vi "DEMO using all functions K_S30_VISA.vi"() -> ()   [LabVIEW 2012]
panel:
  in  "Stopp":bool
  out "Configuration read":u8 format="%.0x"
  in  "Configuration write":u8
  in  "Config. Nr.":u8=1
  in  "Coeff write":sgl format="%.6e"
  out "Coeff read":sgl format="%.6e"
  in  "Coeff. Nr.":u8=64
  out "Status":u8 format="%.0b"
  out "Value":sgl format="%.6e"
  in  "Channel 2":enum16{"CH0", "P1", "P2", "T", "TOB1", "TOB2"}(ring)=enum."P1"
  in  "Target Value":sgl format="%.6e"
  in  "Command":T1(ring)
  in  "F73 read Value":bool
  in  "F33 write config":bool
  in  "F31 write Coeff":bool
  out "Actual Address":u8
  in  "New Address":u8
  out "Serial Nr.":u32
  out "Information":T2
  in  "RS-converter: echo":bool=TRUE
  in  "timeout":u32=50
  in  "Baudrate":enum16{"9600", "115200"}(ring)
  in  "VISA":refnum<visa-resource-name>="COM1"
  in  "F32 read config":bool
  in  "F95 zero":bool
  in  "F66 Device Addr":bool
  in  "F69 SN":bool
  in  "F30 read Coeff":bool
  in  "F48 ini":bool
  in  "Close Com":bool
  in  "Open Com":bool
  in  "Online":bool
  out "error":errorcluster
  out "Value":sgl(graph)
  in  "Channel":enum16{"CH0", "P1", "P2", "T", "TOB1", "TOB2"}(ring)=enum."P1"
  in  "Address":u8=250
  # "Communication with KELLER pressure transmitters Series 3.X using LabView\n\nDemo for all low-level VI's using VISA"
  # "ComPort will also be opened, if you change an parameter for the ComPort"
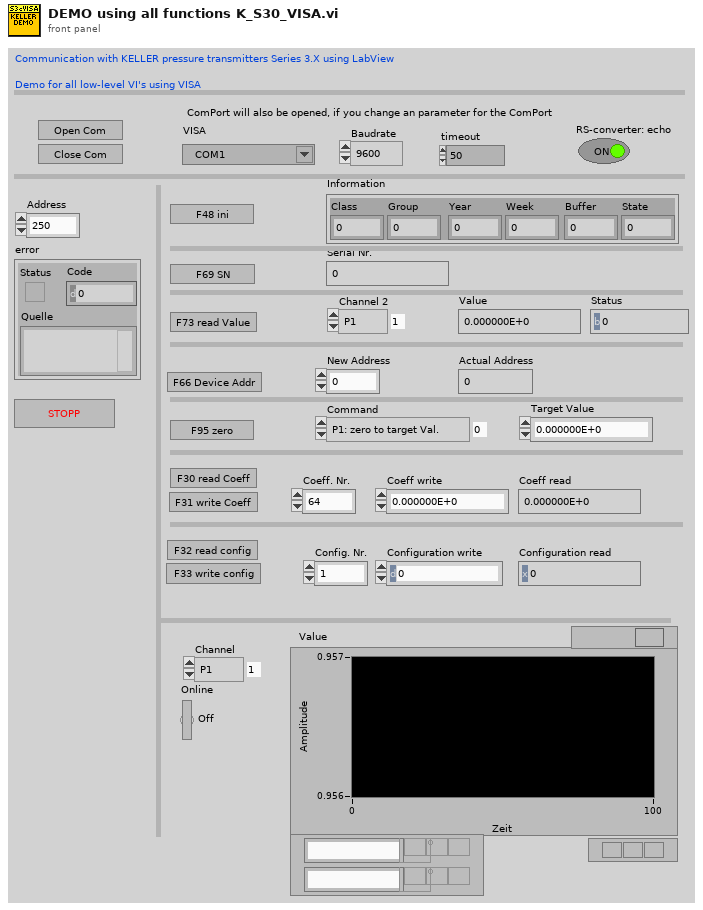
[diagram p1: front panel]
types:
  T1 = enum8{"P1: zero to target Val.", "P1: reset zero", "P2: zero to target Val.", "P2: reset zero", "cmd 4", "cmd 5", "CH0: zero to target Val.", "CH0: reset zero"}
  T2 = cluster{"Class":u8, "Group":u8, "Year":u8, "Week":u8, "Buffer":u8, "State":u8}
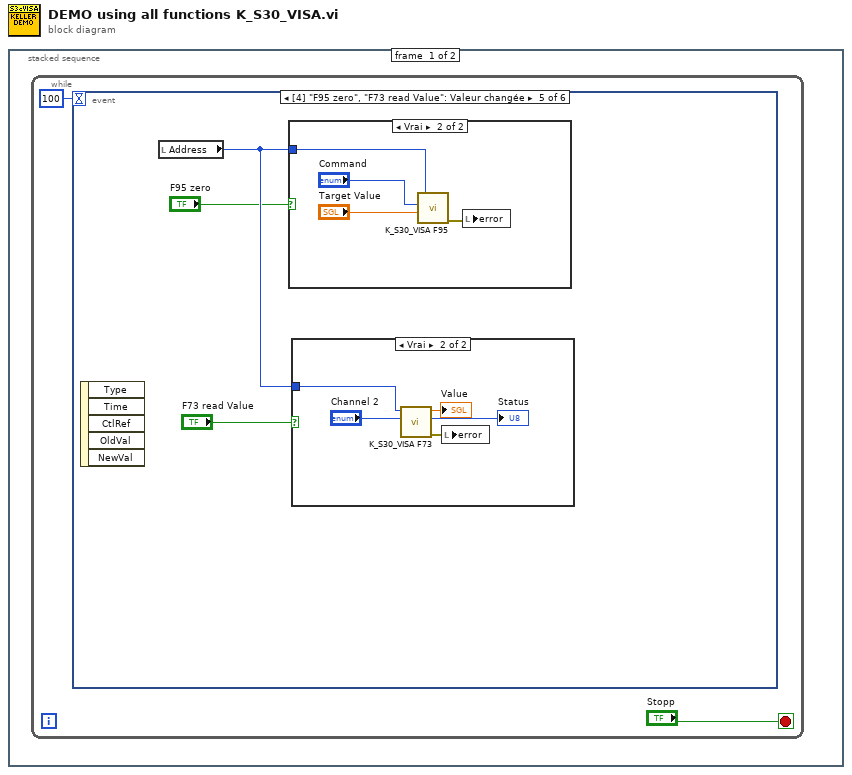
[diagram p0: block diagram]
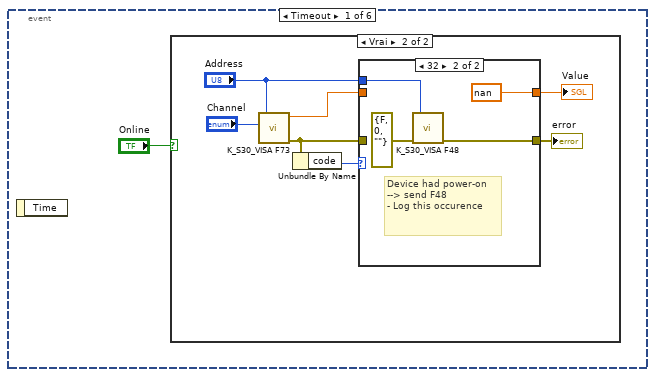
[diagram p2: hidden frame]
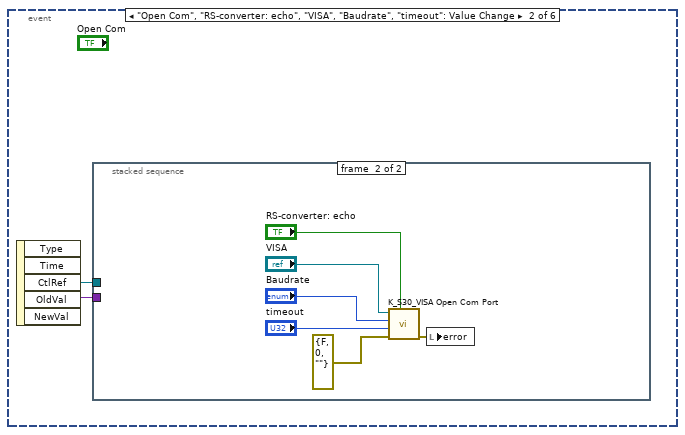
[diagram p5: hidden frame]
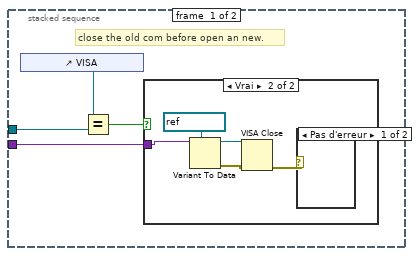
[diagram p6: hidden frame]
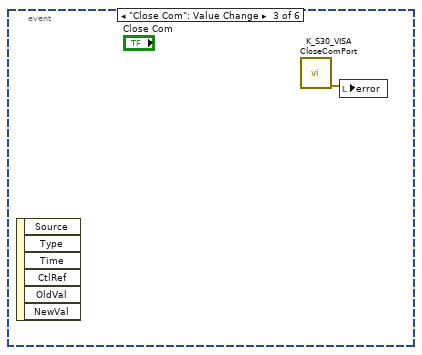
[diagram p9: hidden frame]
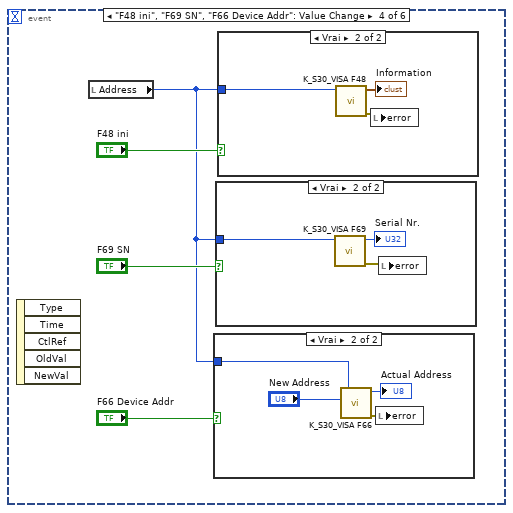
[diagram p10: hidden frame]
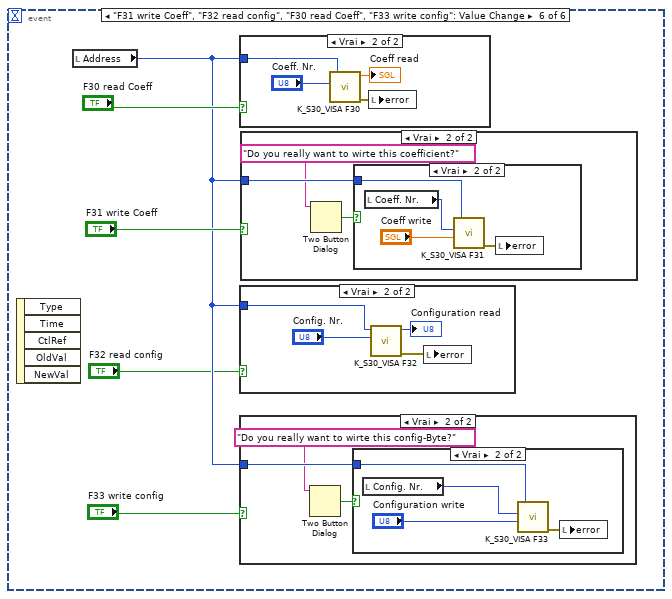
[diagram p16: hidden frame]
diagram:
  n1 = stacked-sequence {
    frame #0 {
      n2 = while {
        stop <- "Stopp" stop-if-true
        n3 = event shown="[4] \"F95 zero\", \"F73 read Value\": Valeur changée" {
          selector: _ -> [_ _ _ _ _ _]
          dyn-events: _ -> [_ _ _ _ _ _]
          timeout: 100 -> [_ _ _ _ _ _]
          event Timeout {
            n4 = event-data() -> ()  [unwired: 1 in, 1 out]
            n5 = case shown="Vrai" "Online" {
              frame False {
              }
              frame True {
                n6 = call "K_S30_VISA F73.vi"("Channel"="Channel", "Address"="Address") -> ("error out"=w7:errorcluster, "Value"=w6:sgl)  [unwired: 3 in, 1 out]
                n7 = Unbundle By Name(w7) -> ("code"=w9:i32)
                n8 = case shown="32" w9 {
                  tunnel: "Address" -> [_ w15]
                  tunnel: w7 -> [w11 _]
                  tunnel: w6 -> [w12 _]
                  tunnel: [w12 sgl nan] -> w5
                  tunnel: [w11 w13] -> w4
                  frame 0, Default {
                  }
                  frame 32 {
                    # "Device had power-on\n--> send F48\n- Log this occurence"
                    n9 = call "K_S30_VISA F48.vi"("error in"=errorcluster {"status"=FALSE, "code"=0, "source"=""}, "Address"=w15) -> ("error out"=w13:errorcluster)  [unwired: 3 in, 2 out]
                  }
                }
                "Value" <- w5
                "error" <- w4
              }
            }
          }
          event "Open Com", "RS-converter: echo", "VISA", "Baudrate", "timeout": Value Change {
            n10 = event-data() -> ("CtlRef"=w18:refnum<vi>, "OldVal"=w17:variant)  [unwired: 1 in, 3 out]
            n11 = stacked-sequence {
              tunnel: w18 -> [w20 _]
              tunnel: w17 -> [w21 _]
              frame #0 {
                # "close the old com before open an new."
                n12 = control-ref of="VISA"() -> (w19:refnum<vi>)
                n13 = Equal?(x=w19, y=w20) -> (x = y?=w22:bool)
                n14 = case shown="Vrai" w22 {
                  tunnel: w21 -> [_ w27]
                  frame False {
                  }
                  frame True {
                    n15 = Variant To Data(type=refnum<visa-resource-name> "COM1" ("VISA resource name"), Variant=w27) -> (data=w25:refnum<visa-resource-name>, error out=w24:errorcluster)  [unwired: 1 in]
                    n16 = VISA Close(VISA resource name=w25, error in (no error)=w24) -> (error out=w23:errorcluster)
                    n17 = case shown="Pas d'erreur" w23 {
                      frame No Error {
                      }
                      frame Error {
                      }
                    }
                  }
                }
              }
              frame #1 {
                n18 = call "K_S30_VISA Open Com Port.vi"("RS-converter:\necho"="RS-converter: echo", "error in (no error)"=errorcluster {"status"=FALSE, "code"=0, "source"=""}, "timeout"="timeout", "Baudrate"="Baudrate", "VISA resource name"="VISA") -> ("error out"=w29:errorcluster)  [unwired: 3 in, 1 out]
                n19 = local write "error"(w29) -> ()
              }
            }
          }
          event "Close Com": Value Change {
            n20 = event-data() -> ()  [unwired: 1 in, 6 out]
            n21 = call "K_S30_VISA CloseComPort.vi"() -> ("Fehlerausgang"=w34:errorcluster)  [unwired: 7 in]
            n22 = local write "error"(w34) -> ()
          }
          event "F48 ini", "F69 SN", "F66 Device Addr": Value Change {
            n23 = event-data() -> ()  [unwired: 1 in, 5 out]
            n24 = local read "Address"() -> (w35:u8)
            n25 = case shown="Vrai" "F66 Device Addr" {
              tunnel: w35 -> [_ w42]
              frame False {
              }
              frame True {
                n26 = call "K_S30_VISA F66.vi"("New Address"="New Address", "Address"=w42) -> ("error out"=w39:errorcluster, "Actual Address"=→"Actual Address":u8)  [unwired: 4 in]
                n27 = local write "error"(w39) -> ()
              }
            }
            n28 = case shown="Vrai" "F69 SN" {
              tunnel: w35 -> [_ w45]
              frame False {
              }
              frame True {
                n29 = call "K_S30_VISA F69.vi"("Address"=w45) -> ("error out"=w43:errorcluster, "Serial Nr."=→"Serial Nr.":u32)  [unwired: 5 in]
                n30 = local write "error"(w43) -> ()
              }
            }
            n31 = case shown="Vrai" "F48 ini" {
              tunnel: w35 -> [_ w46]
              frame False {
              }
              frame True {
                n32 = call "K_S30_VISA F48.vi"("Address"=w46) -> ("error out"=w48:errorcluster, "Information"=→"Information":T2)  [unwired: 4 in, 1 out]
                n33 = local write "error"(w48) -> ()
              }
            }
          }
          event "F95 zero", "F73 read Value": Value Change {
            n34 = event-data() -> ()  [unwired: 1 in, 5 out]
            n35 = local read "Address"() -> (w51:u8)
            n36 = case shown="Vrai" "F95 zero" {
              tunnel: w51 -> [_ w60]
              frame False {
              }
              frame True {
                n37 = call "K_S30_VISA F95.vi"("Target Value"="Target Value", "Command"="Command", "Address"=w60) -> ("error out"=w57:errorcluster)  [unwired: 4 in]
                n38 = local write "error"(w57) -> ()
              }
            }
            n39 = case shown="Vrai" "F73 read Value" {
              tunnel: w51 -> [_ w56]
              frame False {
              }
              frame True {
                n40 = call "K_S30_VISA F73.vi"("Channel"="Channel 2", "Address"=w56) -> ("error out"=w54:errorcluster, "Status"=→"Status":u8, "Value"=→"Value":sgl)  [unwired: 3 in]
                n41 = local write "error"(w54) -> ()
              }
            }
          }
          event "F31 write Coeff", "F32 read config", "F30 read Coeff", "F33 write config": Value Change {
            n42 = event-data() -> ()  [unwired: 1 in, 5 out]
            n43 = local read "Address"() -> (w62:u8)
            n44 = case shown="Vrai" "F30 read Coeff" {
              tunnel: w62 -> [_ w87]
              frame False {
              }
              frame True {
                n45 = call "K_S30_VISA F30.vi"("Coeff. Nr."="Coeff. Nr.", "Address"=w87) -> ("error out"=w85:errorcluster, "Coeff"=→"Coeff read":sgl)  [unwired: 4 in]
                n46 = local write "error"(w85) -> ()
              }
            }
            n47 = case shown="Vrai" "F32 read config" {
              tunnel: w62 -> [_ w76]
              frame False {
              }
              frame True {
                n48 = call "K_S30_VISA F32.vi"("Config. Nr."="Config. Nr.", "Address"=w76) -> ("error out"=w73:errorcluster, "Configuration"=→"Configuration read":u8)  [unwired: 4 in]
                n49 = local write "error"(w73) -> ()
              }
            }
            n50 = case shown="Vrai" "F33 write config" {
              tunnel: w62 -> [_ w68]
              frame False {
              }
              frame True {
                n51 = Two Button Dialog(message="Do you really want to wirte this config-Byte?" ("Nachricht")) -> (T button?=w67:bool)  [unwired: 2 in]
                n52 = case shown="Vrai" w67 {
                  tunnel: w68 -> [_ w72]
                  frame False {
                  }
                  frame True {
                    n53 = local read "Config. Nr."() -> (w70:u8)
                    n54 = call "K_S30_VISA F33.vi"("Configuration"="Configuration write", "Config. Nr."=w70, "Address"=w72) -> ("error out"=w71:errorcluster)  [unwired: 4 in]
                    n55 = local write "error"(w71) -> ()
                  }
                }
              }
            }
            n56 = case shown="Vrai" "F31 write Coeff" {
              tunnel: w62 -> [_ w79]
              frame False {
              }
              frame True {
                n57 = Two Button Dialog(message="Do you really want to wirte this coefficient?" ("Nachricht")) -> (T button?=w78:bool)  [unwired: 2 in]
                n58 = case shown="Vrai" w78 {
                  tunnel: w79 -> [_ w83]
                  frame False {
                  }
                  frame True {
                    n59 = local read "Coeff. Nr."() -> (w82:u8)
                    n60 = call "K_S30_VISA F31.vi"("Coeff. Nr."="Coeff write", "Coeff"=w82, "Address"=w83) -> ("error out"=w80:errorcluster)  [unwired: 4 in]
                    n61 = local write "error"(w80) -> ()
                  }
                }
              }
            }
          }
        }
      }
    }
    frame #1 {
      n62 = call "K_S30_VISA CloseComPort.vi"() -> ()  [unwired: 7 in, 1 out]
    }
  }
